vi "VISA Read.vi"(8 "error in":errorcluster, 10 "Bytes at Port in":u32, 11 "VISA resource in":refnum<visa-resource-name>) -> (0 "error out":errorcluster, 1 "Reading":string, 2 "Bytes at Port out":u32, 3 "VISA resource out":refnum<visa-resource-name>)   [LabVIEW 2021, in "Keysight U1282A.lvlib"]
doc: "Este VI se encarga de realizar la lectura serial con protocolo VISA para el instrumento U1282A, incluso en los modos Trigger Hold y Auto Hold."
uses:
  Keysight U1282A.lvlib
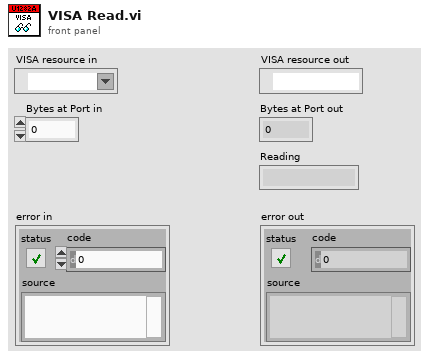
[diagram p1: front panel]
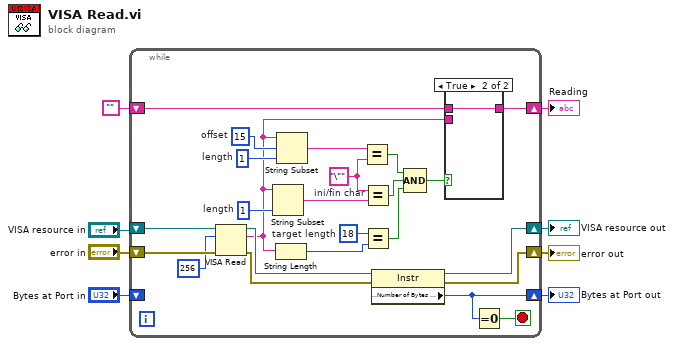
[diagram p0: block diagram]
diagram:
  n1 = while {
    shift-right: [w11] -> w1
    shift-left: "" -> [w12]
    shift-right: [w27] -> w5
    shift-left: "VISA resource in" -> [w9]
    shift-right: [w25] -> w2
    shift-left: "Bytes at Port in" -> [_]
    shift-right: [w26] -> w3
    shift-left: "error in" -> [w31]
    stop <- w32 stop-if-true
    w17 = 18  # target length
    w19 = "\""  # ini/fin char
    w22 = 15  # offset
    w23 = 1  # length
    w24 = 1  # length
    n2 = VISA Read(VISA resource name=w9, byte count=u32 256, error in (no error)=w31) -> (VISA resource name out=w29:refnum<visa-resource-name>, read buffer=w10:string, error out=w28:errorcluster)  [unwired: 1 out]
    n3 = String Subset(string=w10, length (rest)=w24) -> (substring=w20:string)  [unwired: 1 in]
    n4 = String Length(string=w10) -> (length=w18:i32)
    n5 = String Subset(string=w10, offset (0)=w22, length (rest)=w23) -> (substring=w21:string)
    n6 = Equal?(x=w21, y=w19) -> (x = y?=w16:bool)
    n7 = Equal?(x=w19, y=w20) -> (x = y?=w15:bool)
    n8 = Equal?(x=w17, y=w18) -> (x = y?=w14:bool)
    n9 = property class="Instr"(reference=w29, error in=w28) -> (reference out=w27:refnum<visa-resource-name>, error out=w26:errorcluster, "Serial Settings:Number of Bytes at Serial Port"=w25:u32)
    n10 = Compound Arithmetic op=AND(w16, w15, w14) -> (w13:bool)
    n11 = case shown="True" w13 {
      tunnel: w12 -> [_ w34]
      tunnel: w10 -> [w33 _]
      tunnel: [w33 w34] -> w11
      frame False {
      }
      frame True {
      }
    }
    n12 = Equal To 0?(x=w25) -> (x = 0?=w32:bool)
  }
  "VISA resource out" <- w5
  "error out" <- w3
  "Bytes at Port out" <- w2
  "Reading" <- w1
